vi "Create Dir As Needed.vi"(8 "error in (no error)":errorcluster, 11 "Directory In":path) -> (0 "error out":errorcluster, 3 "Directory Out":path)   [LabVIEW 2024]
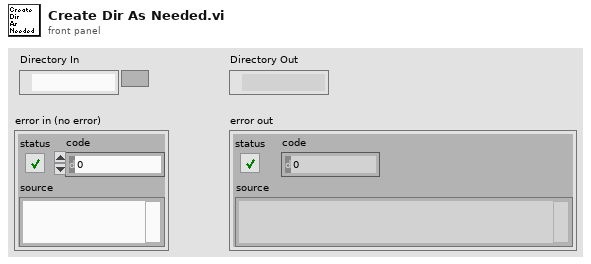
[diagram p1: front panel]
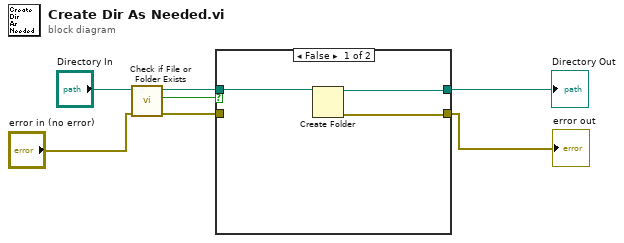
[diagram p0: block diagram]
diagram:
  n1 = call <vilib>:"Check if File or Folder Exists.vi"("error in (no error)"="error in (no error)", "path"="Directory In") -> ("error out"=w3:errorcluster, "file or folder exists?"=w5:bool, "dup path"=w4:path)  [unwired: 7 in]
  n2 = case shown="False" w5 {
    tunnel: w4 -> [w10 w12]
    tunnel: w3 -> [_ w11]
    tunnel: [w9 w12] -> w2
    tunnel: [w8 w11] -> w1
    frame False {
      n3 = Create Folder(path (use dialog)=w10) -> (created path=w9:path, error out=w8:errorcluster)  [unwired: 2 in, 1 out]
    }
    frame True {
    }
  }
  "Directory Out" <- w2
  "error out" <- w1
